vi "Convert U8xU8 to U64.vi"(2 "Input Data":u8[](array[numeric])=[0, 0, 0, 0, 0, 0, 0, 0]) -> (16 "U64":u64)   [LabVIEW 2012]
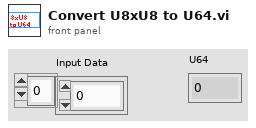
[diagram p1: front panel]
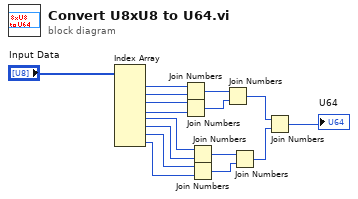
[diagram p0: block diagram]
diagram:
  n1 = Index Array(array="Input Data") -> (element #1=w15:u8, element #2=w16:u8, element #3=w14:u8, element #4=w13:u8, element #5=w4:u8, element #6=w3:u8, element #7=w2:u8, element #8=w1:u8)  [unwired: 8 in]
  n2 = Join Numbers(hi=w15, lo=w16) -> ((hi.lo)=w12:u16)
  n3 = Join Numbers(hi=w14, lo=w13) -> ((hi.lo)=w11:u16)
  n4 = Join Numbers(hi=w4, lo=w3) -> ((hi.lo)=w9:u16)
  n5 = Join Numbers(hi=w2, lo=w1) -> ((hi.lo)=w10:u16)
  n6 = Join Numbers(hi=w12, lo=w11) -> ((hi.lo)=w6:u32)
  n7 = Join Numbers(hi=w9, lo=w10) -> ((hi.lo)=w7:u32)
  n8 = Join Numbers(hi=w6, lo=w7) -> ((hi.lo)=→"U64":u64)
